vi "SQL_SortModifications.vi"(8 "UserLogged":string, 9 "AfterArray":string[](array[string]), 10 "BeforeArray":string[](array[string]), 11 "CleanArray":string[](array[string])) -> (1 "ResultArray":string[](array[string]))   [LabVIEW 2017]
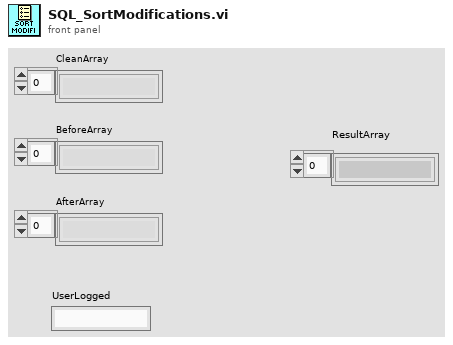
[diagram p1: front panel]
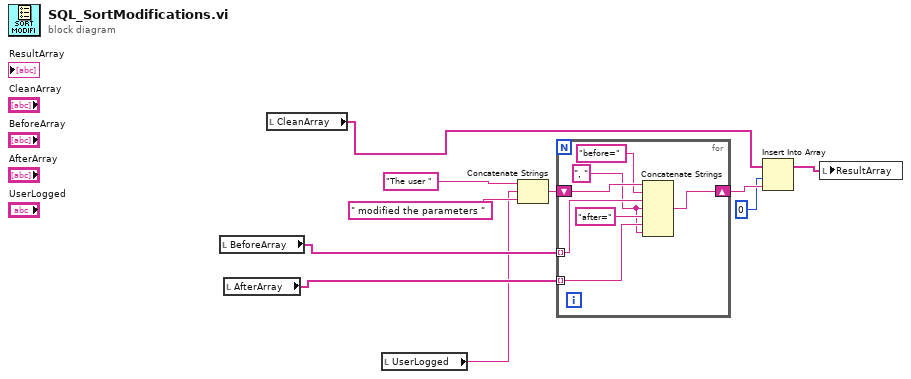
[diagram p0: block diagram]
diagram:
  n1 = local read "BeforeArray"() -> (w3:string[])
  n2 = local read "AfterArray"() -> (w2:string[])
  n3 = local read "CleanArray"() -> (w4:string[])
  n4 = local read "UserLogged"() -> (w1:string)
  n5 = Concatenate Strings("The user ", w1, " modified the parameters ") -> (w8:string)
  n6 = for {
    tunnel: w3 -> [w15] mode=indexing
    tunnel: w2 -> [w13] mode=indexing
    shift-right: [w11] -> w7
    shift-left: w8 -> [w17]
    w12 = ", "
    n7 = Concatenate Strings(w17, "before=", w15, w12, "after=", w13, w12) -> (w11:string)
  }
  n8 = Insert Into Array(array=w4, index=0, new element=w7) -> (w5:string[])
  n9 = local write "ResultArray"(w5) -> ()
